vi "Slot1ConfigurationGlobal.vi"(7 "Action":T3, 11 "Set Value":T1) -> (3 "Value Out":T1)   [LabVIEW 2012]
uses:
  SlotConfigurationGlobalAction.ctl
  SlotConfiguration.ctl
  BankConfiguration.ctl
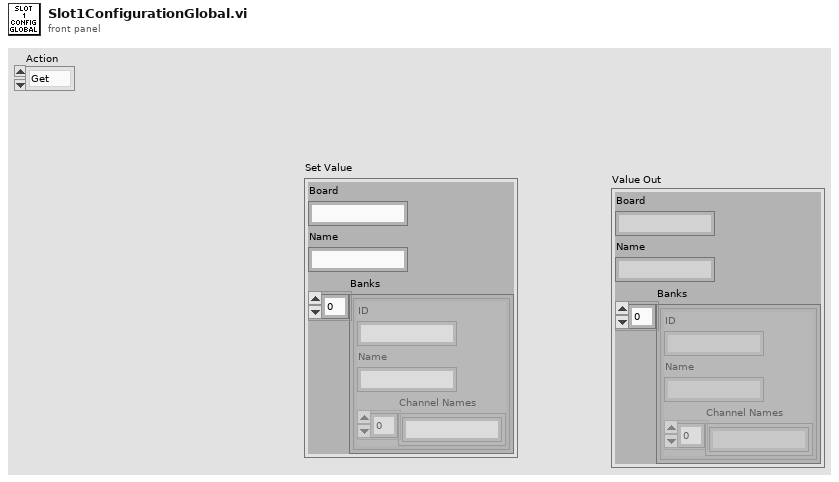
[diagram p1: front panel]
types:
  T1 = typedef "SlotConfiguration.ctl" = cluster{"Board":string, "Name":string, "Banks":T2[]}
  T2 = typedef "BankConfiguration.ctl" = cluster{"ID":string, "Name":string, "Channel Names":string[]}
  T3 = typedef "SlotConfigurationGlobalAction.ctl" = enum16{"Get", "Set", "Reset"}
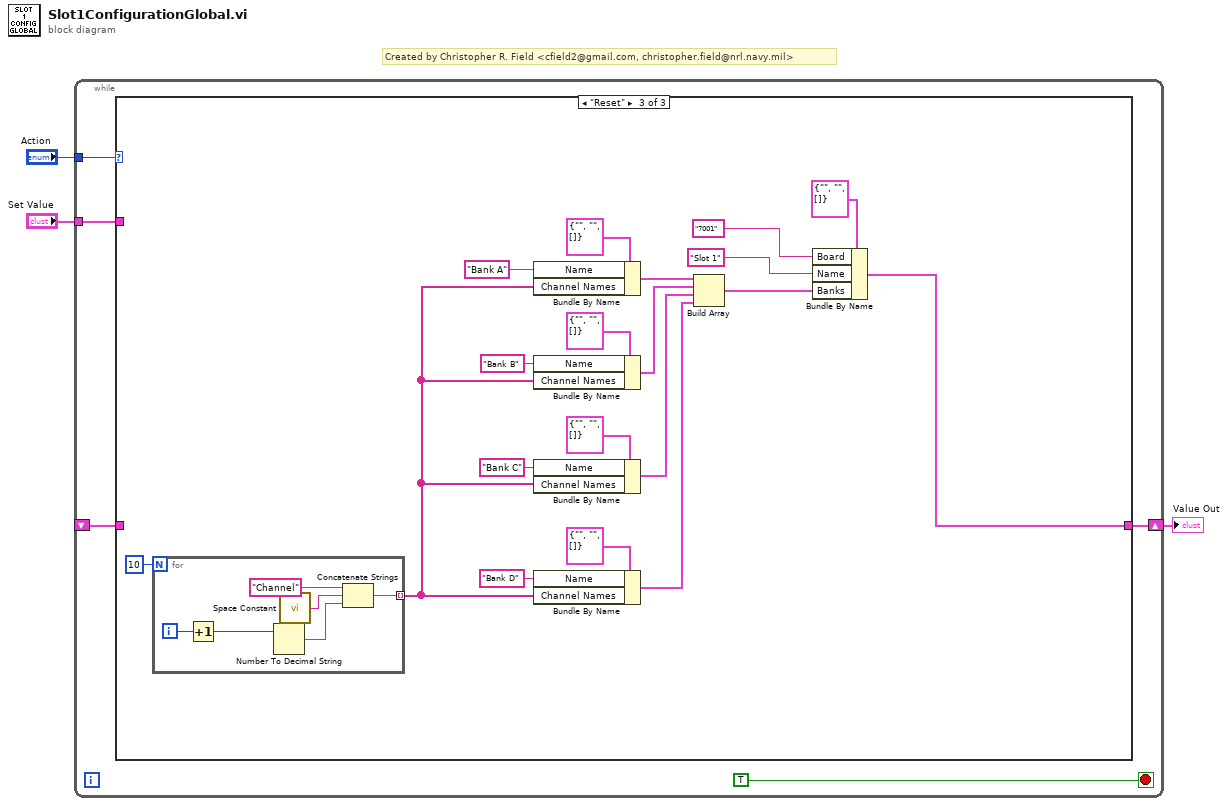
[diagram p0: block diagram]
diagram:
  # "Created by Christopher R. Field <cfield2@gmail.com, christopher.field@nrl.navy.mil>"
  n1 = while {
    tunnel: "Action" -> [w7]
    tunnel: "Set Value" -> [w6]
    shift-right: [w5] -> w1
    shift-left: _ -> [w4]
    stop <- TRUE stop-if-true
    n2 = case shown="\"Reset\"" w7 {
      tunnel: w6 -> [_ w10 _]
      tunnel: [w9 w10 w27] -> w5
      tunnel: w4 -> [w9 _ _]
      frame "Get", Default {
      }
      frame "Set" {
      }
      frame "Reset" {
        n3 = for {
          N: 10 -> [_]
          tunnel: [w30] -> w21 mode=indexing
          i -> [w35]
          n4 = Increment(x=w35) -> (x+1=w34:i32)
          n5 = Number To Decimal String(number=w34) -> (decimal integer string=w31:string)  [unwired: 1 in]
          n6 = call <vilib>:"Space Constant.vi"() -> ("String"=w32:string)
          n7 = Concatenate Strings("Channel", w32, w31) -> (w30:string)
        }
        n8 = Bundle By Name(cluster=T2 {"ID"="", "Name"="", "Channel Names"=[]} ("Bank Configuration"), "Name"="Bank A", "Channel Names"=w21) -> (w17:T2)
        n9 = Bundle By Name(cluster=T2 {"ID"="", "Name"="", "Channel Names"=[]} ("Bank Configuration"), "Name"="Bank B", "Channel Names"=w21) -> (w16:T2)
        n10 = Bundle By Name(cluster=T2 {"ID"="", "Name"="", "Channel Names"=[]} ("Bank Configuration"), "Name"="Bank C", "Channel Names"=w21) -> (w15:T2)
        n11 = Bundle By Name(cluster=T2 {"ID"="", "Name"="", "Channel Names"=[]} ("Bank Configuration"), "Name"="Bank D", "Channel Names"=w21) -> (w14:T2)
        n12 = Build Array(w17, w16, w15, w14) -> (w13:T2[])
        n13 = Bundle By Name(cluster=T1 {"Board"="", "Name"="", "Banks"=[]} ("Slot 1 Configuration"), "Board"="7001", "Name"="Slot 1", "Banks"=w13) -> (w27:T1)
      }
    }
  }
  "Value Out" <- w1
